vi "Double FFT Mesurament Test SLOW.vi"() -> ()   [LabVIEW 2014]
uses:
  <vilib>/Platform/TimedLoop/XDataNode/timing_clust.ctl
  <vilib>/Platform/TimedLoop/XDataNode/nitl_modes.ctl
  <vilib>/Platform/TimedLoop/XDataNode/wakeup.ctl
  <vilib>/rvi/Analysis/measure/FFT/simModelSupport/niFPGA FFT Streaming Sim Properties.ctl
  <vilib>/rvi/Analysis/measure/FFT/simModelSupport/niFPGA FFT Sim Stream Group Properties.ctl
  <vilib>/rvi/Analysis/measure/FFT/simModelSupport/niFPGA FFT Sim Types.ctl
  <vilib>/rvi/Analysis/measure/FFT/simModelSupport/niFpgaFFTSimArithmeticProperties.ctl
  <vilib>/rvi/Analysis/measure/FFT/simModelSupport/niFpgaFFTSimDfxp.ctl
  <vilib>/fxp/LVFixedPointQuantizationPolicyTypeDef.ctl
  <vilib>/rvi/Analysis/measure/FFT/XNode/niFpgaFFTButterflyDelays.ctl
  <vilib>/rvi/Emulation/niFpgaSctlEmulationGetInTimedLoop.vi
  <vilib>/rvi/Emulation/niFpgaEmulationReportErrorSimple.vi
  <vilib>/rvi/Emulation/niFpgaGetClockAttributes.vi
  <vilib>/rvi/Emulation/niFpgaCriticalErrorInLSC.vi
  <vilib>/rvi/Emulation/niFpgaEmulationIsFPGAContextNoSignature.vi
  <vilib>/rvi/DataTransferAndStorage/Container/Common/niFpgaContainerGetUniqueNameForEmu.vi
  <vilib>/rvi/Memory/Memory_Emulation/niFpgaMemoryEmulationCacheClearOnFirstRun.vi
  <vilib>/rvi/Memory/Memory_Emulation/nirvimemoryEmulationManagerCache_MakeExclusive.vi
  <vilib>/rvi/Memory/Memory_Emulation/niFpgaMemoryEmulationValidateCache.vi
  <vilib>/rvi/Memory/Memory_Emulation/nirvimemoryEmulationManagerCache_InsertValue.vi
  <vilib>/Utility/error.llb/Clear Errors.vi
  <vilib>/rvi/Memory/Memory_Emulation/nirvimemoryEmulationManagerCache_ReleaseExclusive.vi
  <vilib>/rvi/Memory/Memory_Emulation/nirvimemoryEmulationManagerCache_GetValue.vi
  <vilib>/rvi/Memory/Memory_Emulation/nirvimemoryEmulationManagerCache_SetValue.vi
  <vilib>/rvi/Emulation/niFpgaProcessEmulError.vi
  <vilib>/rvi/errors/niFpgaSetErrorForExecOnDevCompSimple.vi
  <vilib>/rvi/eio/common/nirviEmuReportErrorAndStop.vi
  <vilib>/rvi/FIFO/Fifo_Resource/nirvififoEmulationSetSize.vi
  <vilib>/rvi/FIFO/Fifo_Resource/nirviFifoEmulationQueueMgr.vi
  <instcachedir>/0/nirviFifoEmulationQueueMgr_E5CAEC123FF24DC58D834DCA3CDAA9B5.lvgen/nirviFifoEmulationQueueMgr_E5CAEC123FF24DC58D834DCA3CDAA9B5_010.vi
  <vilib>/rvi/FIFO/Fifo_Resource/nirvififoEmulationCreateLock.vi
  <vilib>/rvi/FIFO/Fifo_Resource/nirvififoEmulationObtainLock.vi
  <vilib>/rvi/FIFO/Fifo_Resource/nirvififoEmulationReleaseLock.vi
  <vilib>/rvi/occurrence/nirviWaitOnOccurrenceBase.vi
  <vilib>/rvi/errors/nirviReportUnexpectedCaseInternalError.vi
  <vilib>/rvi/errors/nirviReportUnexpectedCaseInternalError (U32).vi
  <vilib>/rvi/FIFO/Fifo_Resource/nirvififoEmulationDetermineInputValidOut.vi
  <vilib>/rvi/Memory/Memory_Emulation/nirvimemoryFastEmulation.vi
  <vilib>/rvi/Memory/Memory_Emulation/nirvimemoryEmulation.vi
  <vilib>/rvi/Analysis/measure/FFT/simModelSupport/niFpgaFFTSimModelStreamingCore.vi
  <vilib>/rvi/interface/RandomDataEmulation/niFpgaRandomDataHandleErrors.vi
  <vilib>/rvi/eio/common/nirviEmuTemplateMethod_errors.vi
  <vilib>/Platform/TimedLoop/XDataNode/XDataNode.xnode
  <vilib>/rvi/DataTransferAndStorage/Container/XNode/niFpgaContainer.xnode
  <vilib>/rvi/DataTransferAndStorage/Register/Emulation/niFpgaRegisterEmulation.vi
  <vilib>/rvi/FIFO/Fifo_Resource/nirvififoEmulationRead.vi
  <vilib>/rvi/FIFO/Fifo_Resource/nirvififoEmulationWrite.vi
  <vilib>/rvi/Analysis/measure/FFT/XNode/niFpgaFFT.xnode
  <vilib>/rvi/interface/RandomDataEmulation/nirviRandomDataFpgaReadWriteTemplate.vi
  <vilib>/eio/EIOMethodNode/EIOMethodNode.xnode
  <vilib>/Platform/TimedLoop/XDataNode/XDNodeRunTimeDep.lvlib
panel:
  in  "Latency points":u32
  in  "snapshot":bool
  in  "lower limit 2":u32=682
  in  "lower limit 1":u32=57
  in  "upper limit 2":u32=1193
  in  "upper limit 1":u32=568
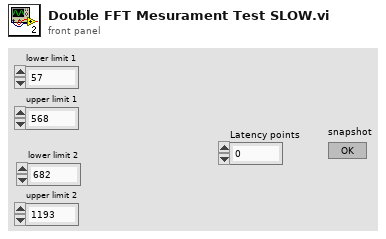
[diagram p1: front panel]
types:
  T1 = typedef "XDNodeRunTimeDep.lvlib/timing_clust.ctl" = cluster{"Expected End [f-1]":u64, "Actual End [f-1]":u64, "Finished Late? [f-1]":bool, "Expected End [i-1]":u64, "Actual End [i-1]":u64, "Finished Late? [i-1]":bool, "Expected Start [i]":u64, "Actual Start [i]":u64, "Expected Start [f]":u64, "Actual Start [f]":u64, "Source Name":string, "Structure Name":string, "Period":i64, "Deadline":i64, "Offset":i64, "Start":i64, "Priority":i32, "Timeout":i32, "Mode":T2, "Wakeup Reason":T3, "Error":errorcluster, "Source Type":string, "Secondary Source Type":string, "Global End Time":u64, "Global Start Time":u64, "Frame Duration":u64, "Iteration Duration":u64, "Assigned CPU":i32, "I/O Scan Engine Mode":u32}
  T2 = typedef "XDNodeRunTimeDep.lvlib/nitl_modes.ctl" = enum32{"No Change", "Process missed periods, maintain original phase", "Discard missed periods, maintain original phase", "Process missed periods, ignore original phase", "Discard missed periods, ignore original phase"}
  T3 = typedef "XDNodeRunTimeDep.lvlib/wakeup.ctl" = enum32{"Normal", "Aborted", "Asynchronous wakeup", "Timing source error", "Timed loop error", "Timeout"}
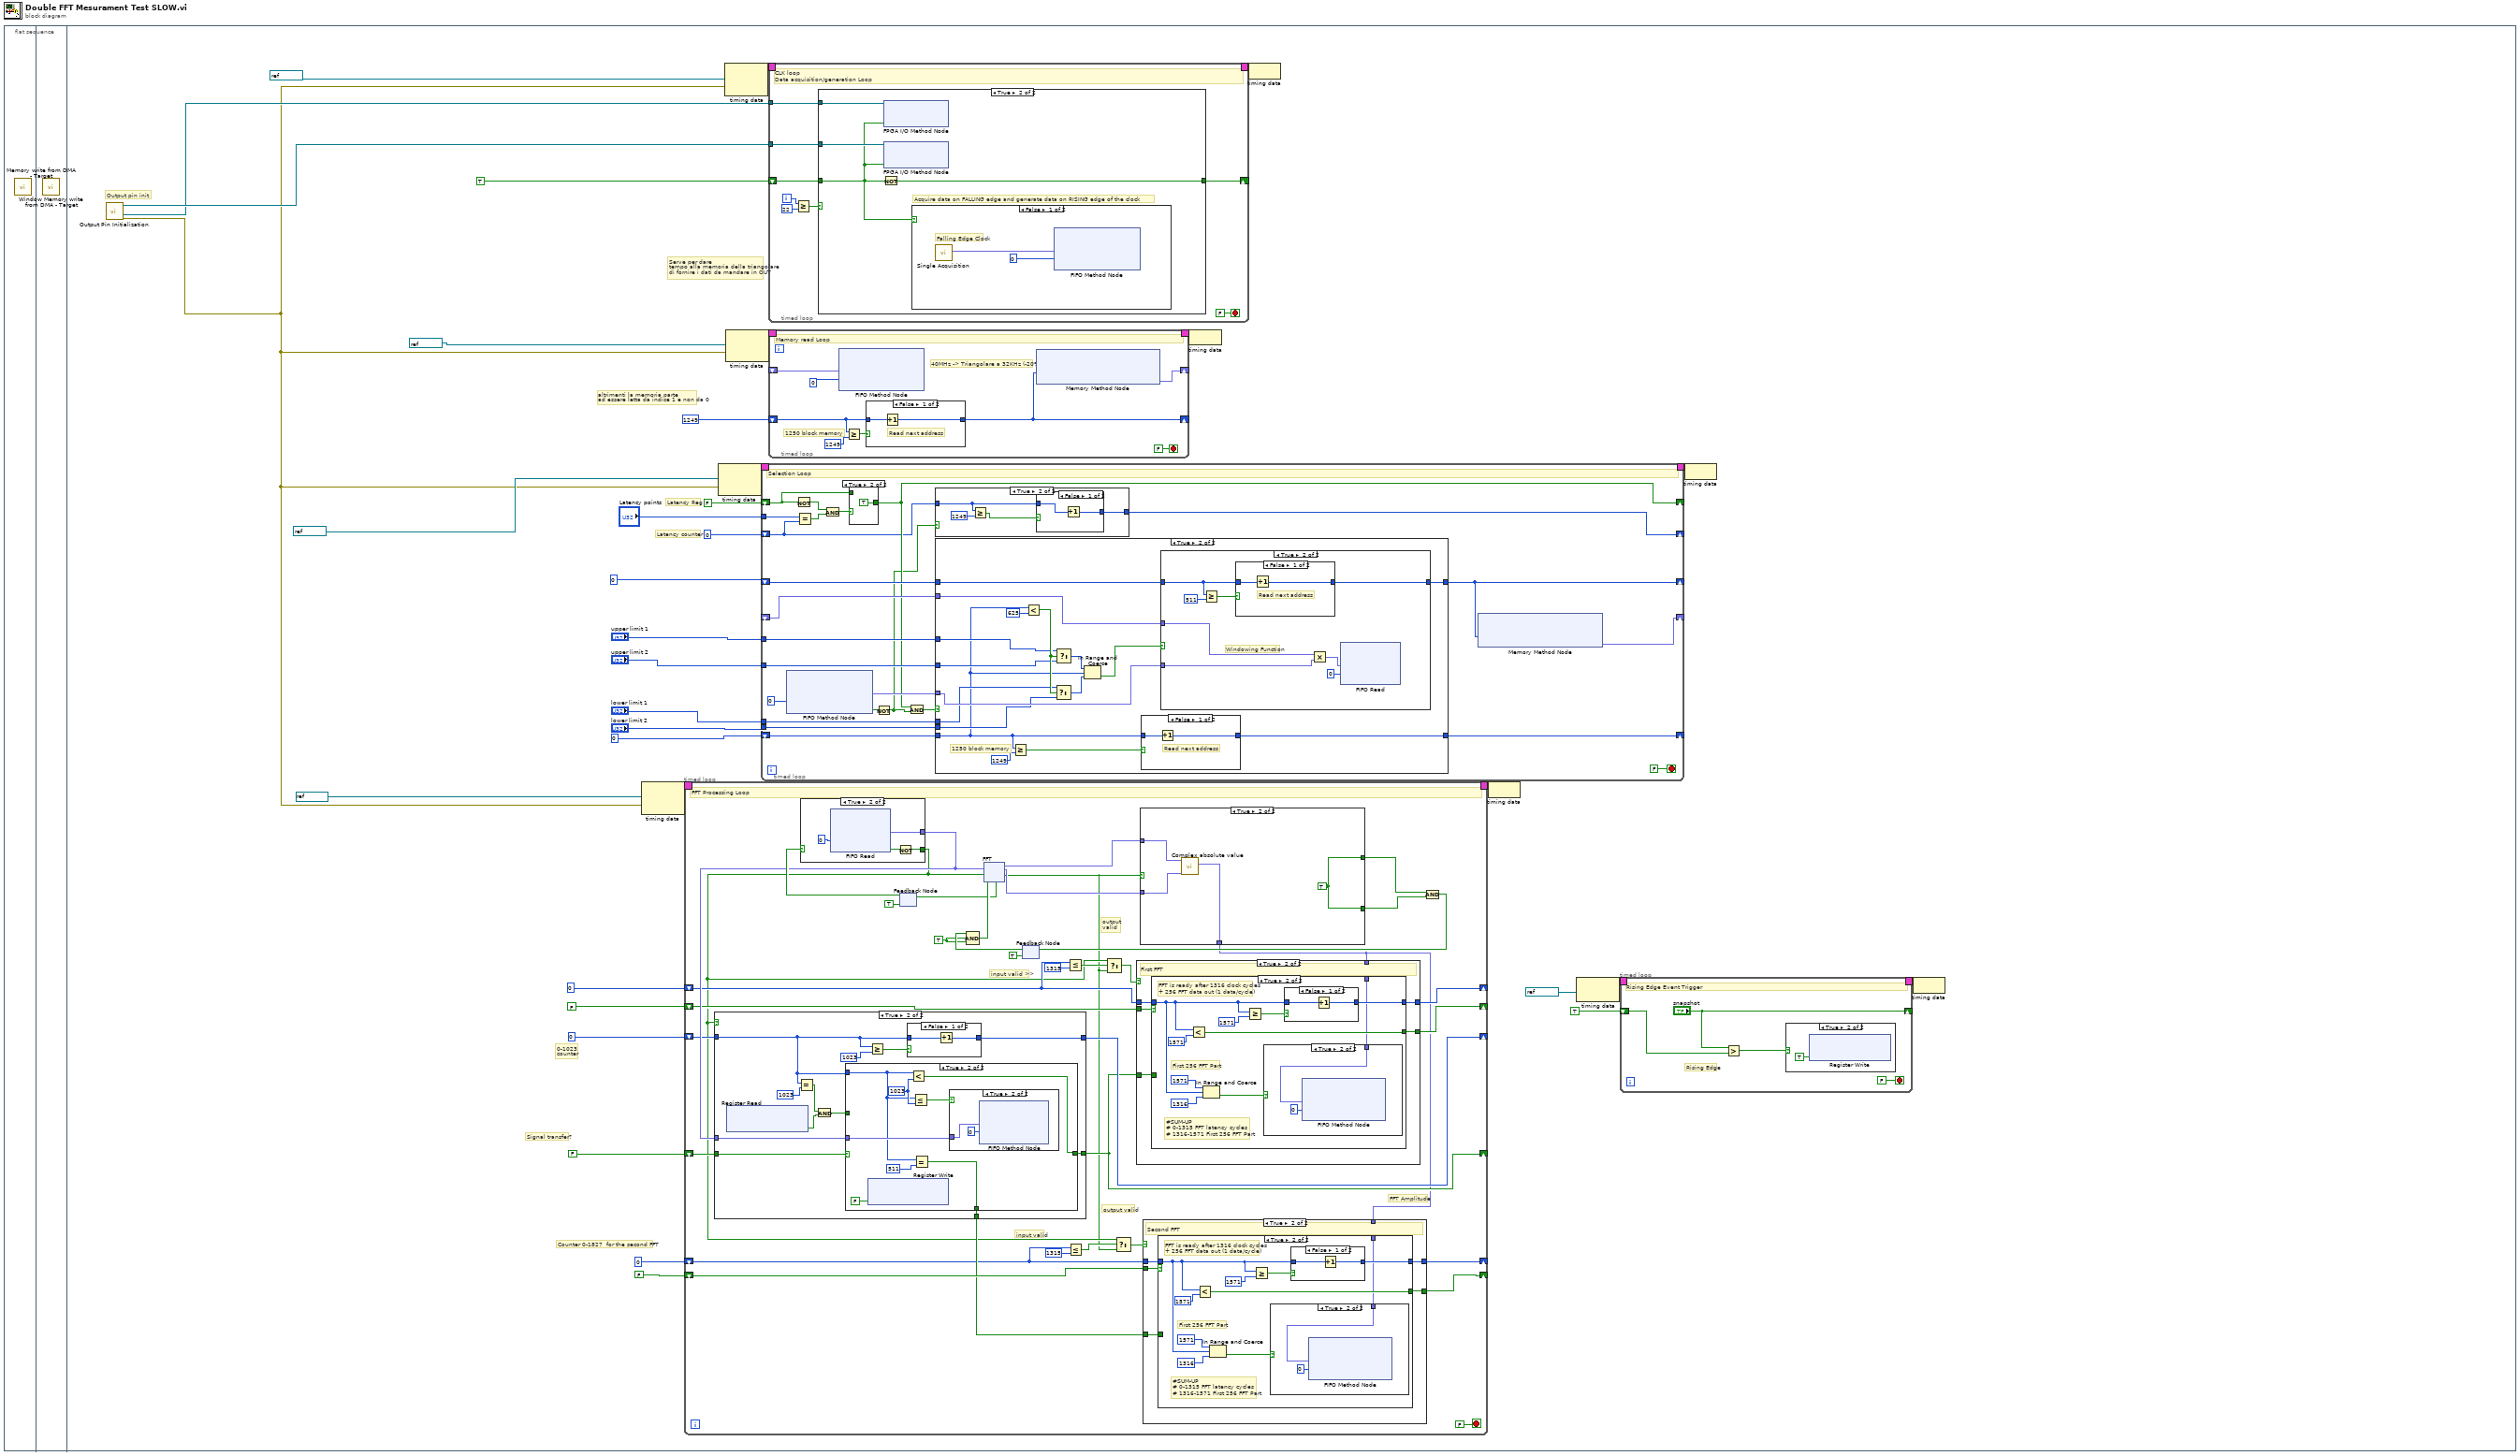
[diagram p0: block diagram]
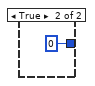
[diagram p4: hidden frame]
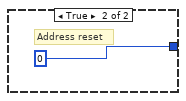
[diagram p8: hidden frame]
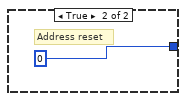
[diagram p9: hidden frame]
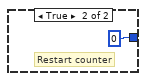
[diagram p13: hidden frame]
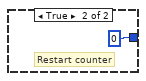
[diagram p17: hidden frame]
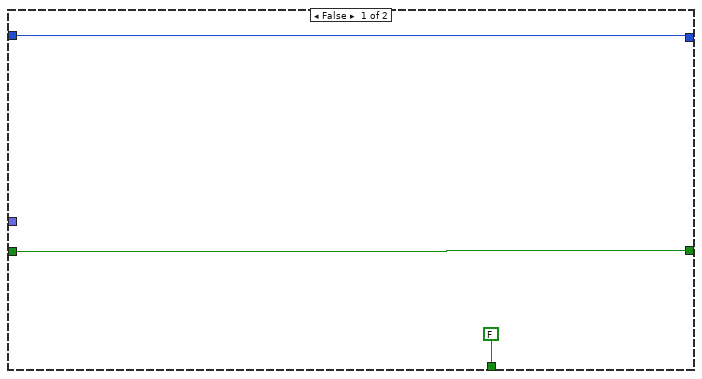
[diagram p18: hidden frame]
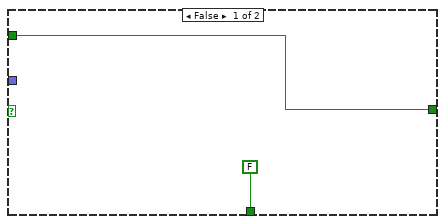
[diagram p19: hidden frame]
diagram:
  n1 = flat-sequence {
    frame #0 {
      n2 = call "Memory write from DMA - Target.vi"() -> ()  [unwired: 12 in]
    }
    frame #1 {
      n3 = call "Window Memory write from DMA - Target.vi"() -> ()  [unwired: 12 in]
    }
    frame #2 {
      # "altrimenti la memoria parte \nad essere letta da indice 1 e non da 0"
      # "Serve per dare\ntempo alla memoria della triangolare\ndi fornire i dati da mandare in OUT"
      # "Latency counter"
      # "Latency Reg"
      # "Counter 0-1827  for the second FFT"
      # "0-1023\ncounter"
      # "Signal transfer?"
      # "Output pin init"
      n4 = call "Output Pin Initialization.vi"() -> ("error out"=w19:errorcluster, "I/O Out Clock DAC (pin16)"=w23:refnum<k21>, "I/O Out Clock ADC (pin17)"=w24:refnum<k21>)  [unwired: 8 in]
      n5 = node-c288(refnum<k21> "30MHz" ("Source Name"), w19) -> (w32:T1)
      n6 = timed-loop {
        timing: w32 -> [_]
        timing-out: [_] -> w31
        shift-right: [w142] -> _
        shift-left: FALSE -> [w145]
        shift-right: [w146] -> _
        shift-left: i16 0 -> [w143]
        shift-right: [w141] -> _
        shift-left: FALSE -> [w140]
        shift-right: [w139] -> _
        shift-left: i16 0 -> [w137]
        shift-right: [w134] -> _
        shift-left: i16 0 -> [w127]
        shift-right: [w131] -> _
        shift-left: FALSE -> [w132]
        stop <- FALSE stop-if-true
        w123 = TRUE
        # "output valid"
        # "input valid"
        # "FFT Amplitude"
        # "output\nvalid"
        # "input valid >>"
        # "FFT Processing Loop"
        n7 = feedback #1(TRUE ("ready for input")) -> (w158:bool)
        n8 = case shown="True" w158 {
          tunnel: [FALSE w275] -> w126
          tunnel: [fxp<+/-,12,12> 0.0 ("Element") w272] -> w144
          frame False {
            # "RMS is not ready for new input"
          }
          frame True {
            n9 = xnode ("FIFO Read")("Timeout"=0) -> ("Element"=w272:fxp<+/-,12,12>, "Timed Out?"=w274:bool)  [unwired: 1 in, 1 out]
            n10 = Not(x=w274) -> (.not. x?=w275:bool)
          }
        }
        n11 = case shown="True" w126 {
          tunnel: w143 -> [w211 w217]
          tunnel: [w211 w221] -> w146
          tunnel: w145 -> [w210 w215]
          tunnel: [w210 w216] -> w142
          tunnel: w144 -> [_ w214]
          tunnel: [FALSE w212] -> w130
          frame False {
          }
          frame True {
            n12 = xnode ("Register Read")() -> ("Data"=w213:bool)  [unwired: 1 in, 1 out]
            n13 = Equal?(x=w217, y=i16 1023) -> (x = y?=w220:bool)
            n14 = And(x=w220, y=w213) -> (x .and. y?=w218:bool)
            n15 = case shown="True" w215 {
              tunnel: w218 -> [w225 _]
              tunnel: w217 -> [_ w228]
              tunnel: [w225 w233] -> w216
              tunnel: w214 -> [_ w231]
              tunnel: [FALSE w226] -> w212
              frame False {
              }
              frame True {
                w230 = i16 1023 ("y")
                n16 = xnode ("Register Write")("Data"=FALSE) -> ()  [unwired: 1 in, 1 out]
                n17 = Less?(x=w228, y=w230) -> (x < y?=w233:bool)
                n18 = Less Or Equal?(x=w228, y=w230) -> (x <= y?=w232:bool)
                n19 = Equal?(x=w228, y=i16 511) -> (x = y?=w226:bool)
                n20 = case shown="True" w232 {
                  tunnel: w231 -> [_ w234]
                  frame False {
                  }
                  frame True {
                    n21 = xnode ("FIFO Method Node")("Element"=w234, "Timeout"=0) -> ()  [unwired: 1 in, 2 out]
                  }
                }
              }
            }
            n22 = Greater Or Equal?(x=w217, y=i16 1023) -> (x >= y?=w222:bool)
            n23 = case shown="False" w222 {
              tunnel: w217 -> [w237 _]
              tunnel: [w236 i16 0] -> w221
              frame False {
                n24 = Increment(x=w237) -> (x+1=w236:i16)
              }
              frame True {
                # "Restart counter"
              }
            }
          }
        }
        n25 = feedback #2(TRUE) -> (w154:bool)
        n26 = Compound Arithmetic op=AND(w154, w123, w123) -> (w153:bool)
        n27 = xnode "FFT"("real data in"=w144, "input valid"=w126, "ready for output"=w153) -> ("ready for input"=w152:bool, "real data out"=w151:fxp<+/-,22,22>, "imaginary data out"=w150:fxp<+/-,22,22>, "output valid"=w124:bool)  [unwired: 2 in, 1 out]
        n28 = feedback-in #1(w152) -> ()
        n29 = Less Or Equal?(x=w137, y=i16 1315) -> (x <= y?=w138:bool)
        n30 = Less Or Equal?(x=w127, y=i16 1315) -> (x <= y?=w128:bool)
        n31 = Select(t=w126, s=w138, f=w124) -> (s? t:f=w135:bool)
        n32 = Select(t=w126, s=w128, f=w124) -> (s? t:f=w125:bool)
        n33 = case shown="True" w124 {
          tunnel: w151 -> [_ w269]
          tunnel: w150 -> [_ w268]
          tunnel: [w265 w266] -> w149
          tunnel: [w265 w266] -> w148
          tunnel: [_ w267] -> w133
          frame False {
            w265 = TRUE
          }
          frame True {
            w266 = TRUE
            n34 = call "Complex absolute value.vi"("Im"=w268, "Re"=w269) -> ("Square Absolute Value"=w267:fxp<+,44,44>)  [unwired: 9 in]
          }
        }
        n35 = case shown="True" w135 {
          tunnel: w142 -> [_ w191]
          tunnel: [w184 w190] -> w141
          tunnel: w140 -> [w184 w189]
          tunnel: w137 -> [w185 w188]
          tunnel: [w185 w187] -> w139
          tunnel: w133 -> [_ w186]
          frame False {
          }
          frame True {
            # "First FFT"
            n36 = case shown="True" w189 {
              tunnel: w191 -> [w193 _]
              tunnel: [w193 w203] -> w190
              tunnel: w188 -> [w192 w196]
              tunnel: [w192 w199] -> w187
              tunnel: w186 -> [_ w194]
              frame False {
              }
              frame True {
                # "First 256 FFT Part"
                # "#SUM-UP\n# 0-1315 FFT latency cycles\n# 1316-1571 First 256 FFT Part"
                # "FFT is ready after 1316 clock cycles\n+ 256 FFT data out (1 data/cycle)"
                n37 = Less?(x=w196, y=i16 1571) -> (x < y?=w203:bool)
                n38 = In Range and Coerce(upper limit=i16 1571, x=w196, lower limit=i16 1316 ("y")) -> (In Range?=w195:bool)  [unwired: 1 out]
                n39 = Greater Or Equal?(x=w196, y=i16 1571) -> (x >= y?=w200:bool)
                n40 = case shown="True" w195 {
                  tunnel: w194 -> [_ w205]
                  frame False {
                  }
                  frame True {
                    n41 = xnode ("FIFO Method Node")("Element"=w205, "Timeout"=0) -> ()  [unwired: 1 in, 2 out]
                  }
                }
                n42 = case shown="False" w200 {
                  tunnel: w196 -> [w207 _]
                  tunnel: [w206 i16 0] -> w199
                  frame False {
                    n43 = Increment(x=w207) -> (x+1=w206:i16)
                  }
                  frame True {
                    # "Restart counter"
                  }
                }
              }
            }
          }
        }
        n44 = case shown="True" w125 {
          tunnel: w130 -> [_ w166]
          tunnel: [w159 w165] -> w131
          tunnel: w132 -> [w159 w164]
          tunnel: w127 -> [w160 w163]
          tunnel: [w160 w162] -> w134
          tunnel: w133 -> [_ w161]
          frame False {
          }
          frame True {
            # "Second FFT"
            n45 = case shown="True" w164 {
              tunnel: w166 -> [w168 _]
              tunnel: [w168 w178] -> w165
              tunnel: w163 -> [w167 w171]
              tunnel: [w167 w174] -> w162
              tunnel: w161 -> [_ w169]
              frame False {
              }
              frame True {
                # "First 256 FFT Part"
                # "#SUM-UP\n# 0-1315 FFT latency cycles\n# 1316-1571 First 256 FFT Part"
                # "FFT is ready after 1316 clock cycles\n+ 256 FFT data out (1 data/cycle)"
                n46 = Less?(x=w171, y=i16 1571) -> (x < y?=w178:bool)
                n47 = In Range and Coerce(upper limit=i16 1571, x=w171, lower limit=i16 1316 ("y")) -> (In Range?=w170:bool)  [unwired: 1 out]
                n48 = Greater Or Equal?(x=w171, y=i16 1571) -> (x >= y?=w175:bool)
                n49 = case shown="True" w170 {
                  tunnel: w169 -> [_ w180]
                  frame False {
                  }
                  frame True {
                    n50 = xnode ("FIFO Method Node")("Element"=w180, "Timeout"=0) -> ()  [unwired: 1 in, 2 out]
                  }
                }
                n51 = case shown="False" w175 {
                  tunnel: w171 -> [w182 _]
                  tunnel: [w181 i16 0] -> w174
                  frame False {
                    n52 = Increment(x=w182) -> (x+1=w181:i16)
                  }
                  frame True {
                    # "Restart counter"
                  }
                }
              }
            }
          }
        }
        n53 = Compound Arithmetic op=AND(w149, w148) -> (w147:bool)
        n54 = feedback-in #2(w147) -> ()
      }
      n55 = node-c288(refnum<k21> "30MHz" ("Source Name"), w19) -> (w30:T1)
      n56 = node-c288(refnum<k21> "60MHz" ("Source Name"), w19) -> (w36:T1)
      n57 = node-c288(refnum<k21> "30MHz" ("Source Name"), w19) -> (w34:T1)
      n58 = timed-loop {
        timing: w30 -> [_]
        timing-out: [_] -> w29
        shift-right: [w70] -> _
        shift-left: u32 0 -> [w57]
        tunnel: "upper limit 1" -> [w66]
        tunnel: "upper limit 2" -> [w65]
        tunnel: "lower limit 1" -> [w64]
        tunnel: "lower limit 2" -> [w63]
        shift-right: [w59] -> _
        shift-left: u32 0 -> [w62]
        shift-right: [w60] -> _
        shift-left: _ -> [w61]
        shift-right: [w51] -> _
        shift-left: FALSE -> [w52]
        tunnel: "Latency points" -> [w56]
        shift-right: [w49] -> _
        shift-left: u32 0 -> [w48]
        stop <- FALSE stop-if-true
        # "Selection Loop"
        n59 = xnode ("FIFO Method Node")("Timeout"=0) -> ("Element"=w68:fxp<+/-,12,12>, "Timed Out?"=w69:bool)  [unwired: 1 in, 1 out]
        n60 = Not(x=w52) -> (.not. x?=w55:bool)
        n61 = Equal?(x=w56, y=w48) -> (x = y?=w54:bool)
        n62 = And(x=w55, y=w54) -> (x .and. y?=w53:bool)
        n63 = case shown="True" w53 {
          tunnel: [w80 TRUE] -> w51
          tunnel: w52 -> [w80 _]
          frame False {
          }
          frame True {
          }
        }
        n64 = Not(x=w69) -> (.not. x?=w50:bool)
        n65 = And(x=w51, y=w50) -> (x .and. y?=w58:bool)
        n66 = case shown="True" w50 {
          tunnel: w48 -> [w72 w75]
          tunnel: [w72 w73] -> w49
          frame False {
          }
          frame True {
            n67 = Greater Or Equal?(x=w75, y=u32 1249) -> (x >= y?=w74:bool)
            n68 = case shown="False" w74 {
              tunnel: w75 -> [w78 _]
              tunnel: [w77 u32 0] -> w73
              frame False {
                n69 = Increment(x=w78) -> (x+1=w77:u32)
              }
              frame True {
              }
            }
          }
        }
        n70 = case shown="True" w58 {
          tunnel: [w83 w98] -> w70
          tunnel: w57 -> [w83 w85]
          tunnel: w68 -> [_ w93]
          tunnel: w66 -> [_ w92]
          tunnel: w65 -> [_ w91]
          tunnel: w64 -> [_ w90]
          tunnel: w63 -> [_ w89]
          tunnel: w62 -> [w82 w86]
          tunnel: [w82 w88] -> w59
          tunnel: w61 -> [_ w87]
          frame False {
          }
          frame True {
            # "1250 block memory"
            n71 = Greater Or Equal?(x=w85, y=u32 1249) -> (x >= y?=w99:bool)
            n72 = Less?(x=w85, y=u32 625) -> (x < y?=w94:bool)
            n73 = Select(t=w90, s=w94, f=w89) -> (s? t:f=w96:u32)
            n74 = Select(t=w92, s=w94, f=w91) -> (s? t:f=w97:u32)
            n75 = In Range and Coerce(upper limit=w97, x=w85, lower limit=w96) -> (In Range?=w84:bool)  [unwired: 1 out]
            n76 = case shown="False" w99 {
              tunnel: w85 -> [w114 _]
              tunnel: [w113 u32 0] -> w98
              frame False {
                # "Read next address"
                n77 = Increment(x=w114) -> (x+1=w113:u32)
              }
              frame True {
                # "Address reset"
              }
            }
            n78 = case shown="True" w84 {
              tunnel: w93 -> [_ w102]
              tunnel: w86 -> [w101 w107]
              tunnel: [w101 w109] -> w88
              tunnel: w87 -> [_ w105]
              frame False {
              }
              frame True {
                # "Windowing Function"
                n79 = Greater Or Equal?(x=w107, y=u32 511) -> (x >= y?=w108:bool)
                n80 = case shown="False" w108 {
                  tunnel: w107 -> [w111 _]
                  tunnel: [w110 u32 0] -> w109
                  frame False {
                    # "Read next address"
                    n81 = Increment(x=w111) -> (x+1=w110:u32)
                  }
                  frame True {
                    # "Address reset"
                  }
                }
                n82 = Multiply(x=w105, y=w102) -> (x*y=w103:fxp<+/-,12,12>)
                n83 = xnode ("FIFO Read")("Element"=w103, "Timeout"=0) -> ()  [unwired: 1 in, 2 out]
              }
            }
          }
        }
        n84 = xnode ("Memory Method Node")("Address"=w59) -> ("Data"=w60:fxp<+,8,1>)  [unwired: 1 in, 1 out]
      }
      n85 = timed-loop {
        timing: w36 -> [_]
        timing-out: [_] -> w35
        shift-right: [w306] -> _
        shift-left: TRUE -> [w304]
        tunnel: w23 -> [w308]
        tunnel: w24 -> [w305]
        i -> [w302]
        stop <- FALSE stop-if-true
        # "CLK loop\nData acquisition/generation Loop"
        n86 = Greater Or Equal?(x=w302, y=22) -> (x >= y?=w301:bool)
        n87 = case shown="True" w301 {
          tunnel: w308 -> [_ w313]
          tunnel: [w309 w312] -> w306
          tunnel: w305 -> [_ w311]
          tunnel: w304 -> [w309 w310]
          frame False {
          }
          frame True {
            # "Acquire data on FALLING edge and generate data on RISING edge of the clock"
            n88 = Not(x=w310) -> (.not. x?=w312:bool)
            n89 = xnode "FPGA I/O Method Node"("FPGA I/O In"=w313, "Data"=w310) -> ()  [unwired: 1 out]
            n90 = xnode "FPGA I/O Method Node"("FPGA I/O In"=w311, "Data"=w310) -> ()  [unwired: 1 out]
            n91 = case shown="False" w310 {
              frame False {
                # "Falling Edge Clock"
                n92 = call "Single Acquisition.vi"() -> ("Out"=w315:fxp<+/-,12,12>)  [unwired: 10 in, 1 out]
                n93 = xnode ("FIFO Method Node")("Element"=w315, "Timeout"=0) -> ()  [unwired: 1 in, 2 out]
              }
              frame True {
                # "Rising Edge Clock"
                n94 = xnode ("FIFO Method Node")("Timeout"=0) -> ("Element"=w316:fxp<+/-,12,12>, "Timed Out?"=w317:bool)  [unwired: 1 in, 1 out]
                n95 = case shown="False" w317 {
                  tunnel: w316 -> [w321 _]
                  frame False {
                    # "Data Generation"
                    n96 = Add(x=w321, y=fxp<+,12,12> 2048.0) -> (x+y=w319:fxp<+/-,14,14>)
                    n97 = call "Single Point Wave generation.vi"("Data To Write"=w319) -> ()  [unwired: 10 in, 1 out]
                  }
                  frame True {
                    # "FPGA memory slow"
                  }
                }
              }
            }
          }
        }
      }
      n98 = timed-loop {
        timing: w34 -> [_]
        timing-out: [_] -> w33
        shift-right: [w283] -> _
        shift-left: u32 1249 -> [w287]
        shift-right: [w285] -> _
        shift-left: _ -> [w284]
        stop <- FALSE stop-if-true
        # "40MHz -> Triangolare a 32KHz (-20%)"
        # "1250 block memory"
        # "Memory read Loop"
        n99 = xnode ("FIFO Method Node")("Element"=w284, "Timeout"=0) -> ()  [unwired: 1 in, 2 out]
        n100 = Greater Or Equal?(x=w287, y=u32 1249) -> (x >= y?=w289:bool)
        n101 = case shown="False" w289 {
          tunnel: w287 -> [w292 _]
          tunnel: [w291 u32 0] -> w283
          frame False {
            # "Read next address"
            n102 = Increment(x=w292) -> (x+1=w291:u32)
          }
          frame True {
            # "Address reset"
          }
        }
        n103 = xnode ("Memory Method Node")("Address"=w283) -> ("Data"=w285:fxp<+/-,12,12>)  [unwired: 1 in, 1 out]
      }
      n104 = node-c288(w33) -> ()
      n105 = node-c288(w35) -> ()
      n106 = node-c288(w31) -> ()
      n107 = node-c288(refnum<k21> "30MHz" ("Source Name")) -> (w9:T1)
      n108 = timed-loop {
        timing: w9 -> [_]
        timing-out: [_] -> w8
        shift-right: ["snapshot"] -> _
        shift-left: TRUE ("snapshot") -> [w39]
        stop <- FALSE stop-if-true
        # "Rising Edge"
        # "Rising Edge Event Trigger"
        n109 = Greater?(x="snapshot", y=w39) -> (0:w37:bool)
        n110 = case shown="True" w37 {
          frame False {
          }
          frame True {
            n111 = xnode ("Register Write")("Data"=TRUE) -> ()  [unwired: 1 in, 1 out]
          }
        }
      }
      n112 = node-c288(w29) -> ()
      n113 = node-c288(w8) -> ()
    }
  }
